vi "Add Manager Error Core.vi"(8 "error in (no error)":errorcluster, 10 "String to Append":string, 11 "Error":T1) -> (0 "error out":errorcluster)   [LabVIEW 2021, in "Manager Common.lvlib"]
uses:
  Manager Common.lvlib
  typedef/Manager Errors.ctl
  <vilib>/CIF Foundation/CIF Utilities/Errors/Errors_CIF_U.lvlib
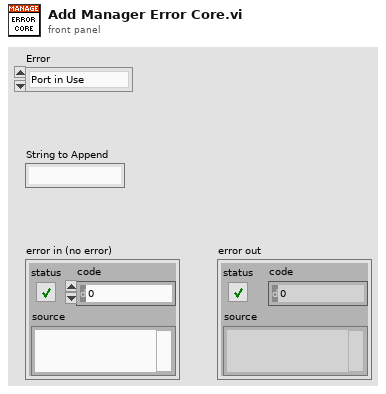
[diagram p1: front panel]
types:
  T1 = typedef "Manager Common.lvlib/Manager Errors.ctl" = enum16{"Port in Use"}
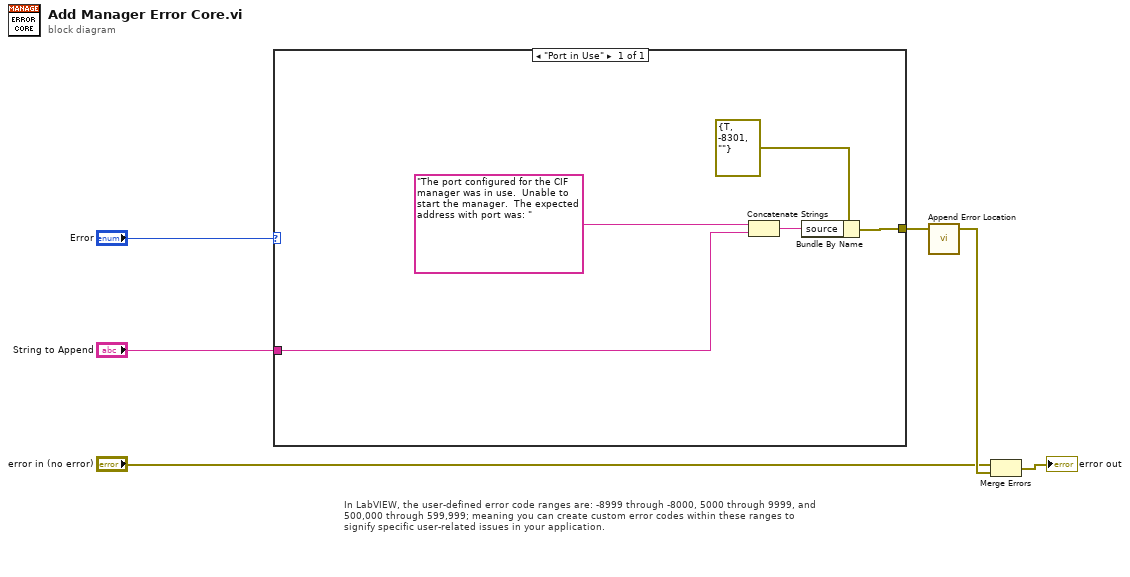
[diagram p0: block diagram]
diagram:
  # "In LabVIEW, the user-defined error code ranges are: -8999 through -8000, 5000 through 9999, and 500,000 through 599,999; meaning you can create custom error codes within these ranges to signify specific user-related issues in your application."
  n1 = case shown="\"Port in Use\"" "Error" {
    tunnel: "String to Append" -> [w8]
    tunnel: [w10] -> w5
    frame "Port in Use" {
      n2 = Concatenate Strings("The port configured for the CIF manager was in use.  Unable to start the manager.  The expected address with port was: " ("source"), w8) -> (w7:string)
      n3 = Bundle By Name(cluster=errorcluster {"status"=TRUE, "code"=-8301, "source"=""} ("Invalid ID"), "source"=w7) -> (w10:errorcluster)
    }
  }
  n4 = call <vilib>:"Append Error Location.vi"("error in (no error)"=w5) -> ("error out"=w6:errorcluster)  [unwired: 4 in]
  n5 = Merge Errors("error in (no error)", w6) -> (→"error out":errorcluster)
